vi "Acquire_EnergyCalibrationCurve.vi"(11 "Queue in":refnum<queue>) -> (2 "Angle-Energy Cali. Curve":cluster{dbl[], dbl[]}(graph))   [LabVIEW 2013]
uses:
  <instrlib>/ESP300/Public/Data/ESP300_State.ctl
  <instrlib>/ESP300/Public/Position_ESP300.vi
  ControlDef/MiscParams.vi
  <userlib>/_OpenG.lib/comparison/comparison.llb/DBL Changed__ogtk.vi
  <instrlib>/ESP300/ESP300.lvlib
panel:
  in  "stop":bool
  out "Percentage":dbl
  out "Energy Cali. Array":cluster{"Angle":dbl, "Energy":dbl}[](array[cluster])
  out "Current Energy":dbl
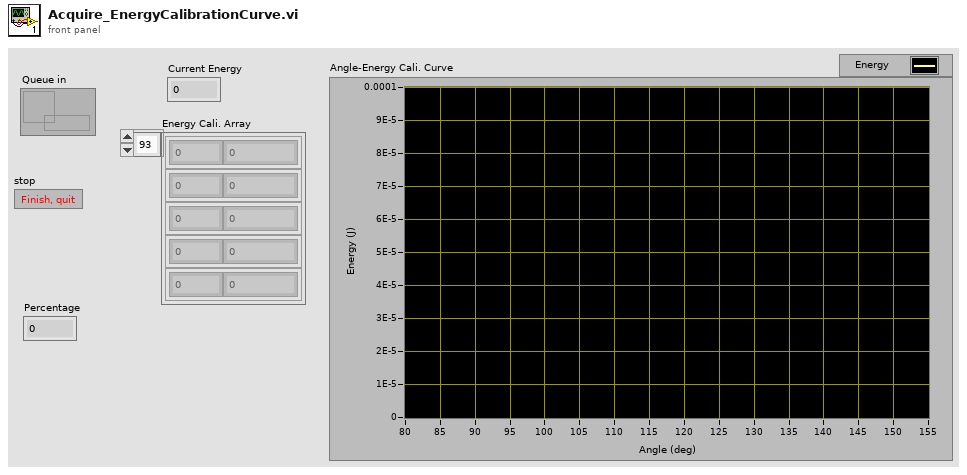
[diagram p1: front panel]
types:
  T1 = typedef "ESP300.lvlib/ESP300_State.ctl" = cluster{"State":enum16{"Initialize", "SetDefaultConfig", "Close", "Quit", "Identify", "MoveAbs", "MoveAbs_all", "MoveRel", "MoveRel_all", "STOP", "Origin/Home", "WaitStop", "QueryStatus", "UpdateXPos", "UpdateAll", "SetVelocity", "SetAcceleration", "ClearErr", "LogMessage", "MotorEnable(1)", "EnableAxis", "JoyStick", "GetVelocity", "GetAcceleration", "SendCmd", "SetSoftLimits", "Beep", "_SettingReturn", "SoftReset"}, "Params.":variant}
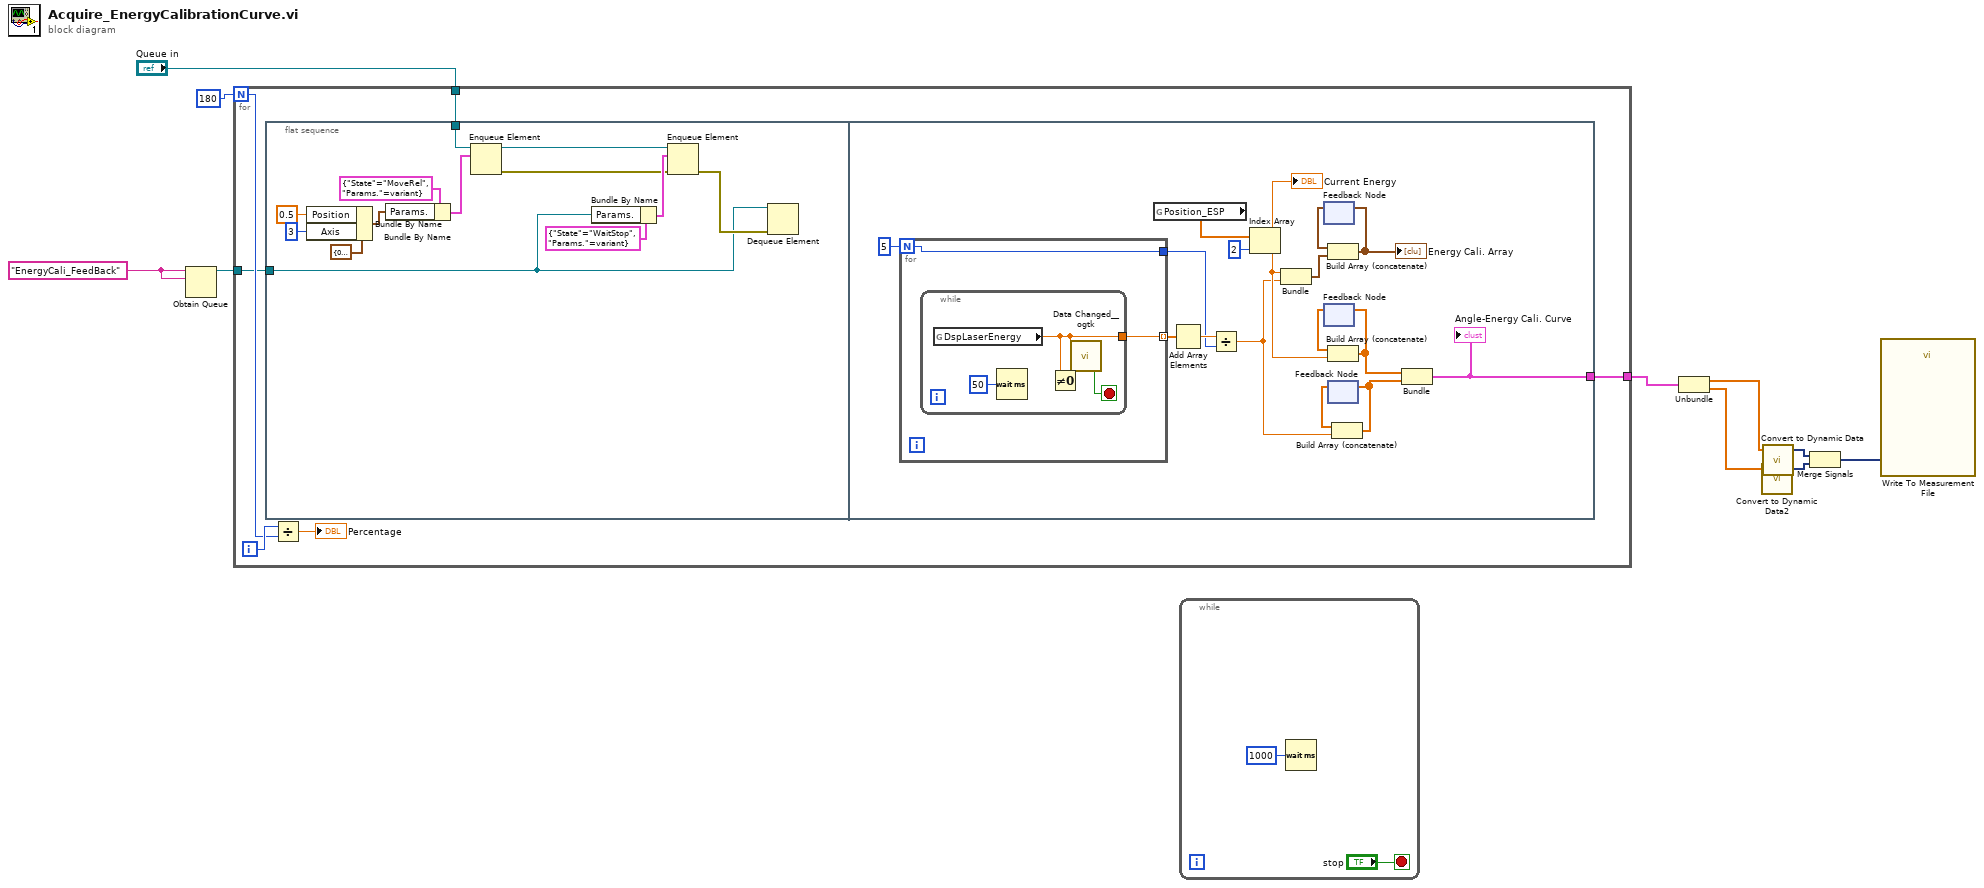
[diagram p0: block diagram]
diagram:
  w8 = "EnergyCali_FeedBack" ("name (unnamed)")
  n1 = Obtain Queue(name (unnamed)=w8, element data type=w8) -> (queue out=w7:refnum<queue>)  [unwired: 3 in, 2 out]
  n2 = for {
    N: 180 -> [w14]
    tunnel: "Queue in" -> [w16]
    tunnel: w7 -> [w13]
    tunnel: [w11] -> w6
    i -> [w15]
    n3 = flat-sequence {
      tunnel: w16 -> [w23]
      tunnel: w13 -> [w18]
      tunnel: [w30] -> w11
      frame #0 {
        n4 = Bundle By Name(cluster=cluster{"Axis":i32, "Position":dbl} {"Axis"=0, "Position"=0.0}, "Position"=0.5, "Axis"=3) -> (w29:cluster{"Axis":i32, "Position":dbl})
        n5 = Bundle By Name(cluster=T1 {"State"=enum."MoveRel", "Params."=variant} ("element"), "Params."=w29) -> (w24:T1)
        n6 = Enqueue Element(queue=w23, element=w24) -> (queue out=w17:refnum<queue>, error out=w19:errorcluster)  [unwired: 2 in, 1 out]
        n7 = Bundle By Name(cluster=T1 {"State"=enum."WaitStop", "Params."=variant} ("element"), "Params."=w18) -> (w21:T1)
        n8 = Enqueue Element(queue=w17, element=w21, error in (no error)=w19) -> (error out=w22:errorcluster)  [unwired: 1 in, 2 out]
        n9 = Dequeue Element(queue=w18, error in (no error)=w22) -> ()  [unwired: 1 in, 4 out]
      }
      frame #1 {
        n10 = for {
          N: 5 -> [w46]
          tunnel: [w47] -> w35 mode=indexing
          tunnel: [w46] -> w33
          n11 = while {
            tunnel: [w49] -> w47
            stop <- w48 stop-if-true
            n12 = global read "MiscParams.vi" "DspLaserEnergy"() -> (w49:dbl)
            n13 = Wait (ms)(milliseconds to wait=u32 50) -> ()  [unwired: 1 out]
            n14 = Not Equal To 0?(x=w49) -> ()  [unwired: 1 out]
            n15 = call-poly <userlib>:"Data Changed__ogtk.vi"("DBL"=w49) -> ("Changed"=w48:bool)
          }
        }
        n16 = global read "Position_ESP300.vi" "Position_ESP"() -> (w44:dbl[])
        n17 = Add Array Elements(numeric array=w35) -> (sum=w34:dbl)
        n18 = Divide(x=w34, y=w33) -> (x/y=w32:dbl)
        n19 = Index Array(array=w44, index=2) -> (element=w40:dbl)
        "Current Energy" <- w40
        n20 = Bundle(w40, w32) -> (w37:cluster{dbl, dbl})  [unwired: 1 in]
        n21 = feedback #1() -> (w45:cluster{dbl, dbl}[])  [unwired: 1 in]
        n22 = feedback #2() -> (w42:dbl[])  [unwired: 1 in]
        n23 = Build Array (concatenate)(w45, w37) -> (w43:cluster{dbl, dbl}[])
        "Energy Cali. Array" <- w43
        n24 = feedback-in #1(w43) -> ()
        n25 = Build Array (concatenate)(w42, w40) -> (w39:dbl[])
        n26 = feedback-in #2(w39) -> ()
        n27 = feedback #3() -> (w41:dbl[])  [unwired: 1 in]
        n28 = Build Array (concatenate)(w41, w32) -> (w38:dbl[])
        n29 = feedback-in #3(w38) -> ()
        n30 = Bundle(w39, w38) -> (w30:cluster{dbl[], dbl[]})  [unwired: 1 in]
        "Angle-Energy Cali. Curve" <- w30
      }
    }
    n31 = Divide(x=w15, y=w14) -> (x/y=→"Percentage":dbl)
  }
  n32 = while {
    stop <- "stop" stop-if-true
    n33 = Wait (ms)(milliseconds to wait=u32 1000) -> ()  [unwired: 1 out]
  }
  n34 = Unbundle(w6) -> (w5:dbl[], w4:dbl[])
  n35 = call "Convert to Dynamic Data2"("Array"=w4) -> ("Dynamic Data Type"=w2:dynamicdata)  [unwired: 3 in]
  n36 = call "Convert to Dynamic Data"("Array"=w5) -> ("Dynamic Data Type"=w3:dynamicdata)  [unwired: 3 in]
  n37 = Merge Signals(w3, w2) -> (w1:dynamicdata)
  n38 = call "Write To Measurement File"("Signals"=w1) -> ()  [unwired: 16 in, 3 out]
